vi "SW_Gen_Get_Initial_picture_Scaling_and_Cage_size.vi"(8 "Input cluster of parameters":T2={"Amount of border segments"=8, "Border segments starting angle"=0, "Amount of midfield segments"=4, "Midfield segments starting angle"=0, "Midfield segments outer radius, mm"=60, "Amount of central segments"=1, "Center segment outer radius, mm"=30, "Diameter of the cage, mm"=180, "R-gap between segments, mm"=10} {"Diameter of the cage, mm" scale=20.0..250.0}, 9 "Scale factor for outer display radius display":dbl=0.95 format="%#_13g", 10 "Background color":u32(colorbox)=13816530, 11 "Draw Area Size":cluster{"Width":dbl, "Height":dbl}={"Width"=480.0, "Height"=480.0}) -> (0 "Cluster of image geometrical and scaling parameters":T1, 3 "Zones display background":picture)   [LabVIEW 2018, in "Tracker.lvlib"]
uses:
  Tracker.lvlib
panel:
  out "Radius of displayed central segment, pix":dbl
  out "Radius of displayed midfield segments, pix":dbl
  out "Pixels per mm":dbl
  out "Radius of displayed outer segments, pix":dbl
  out "Fonts scale factor":dbl
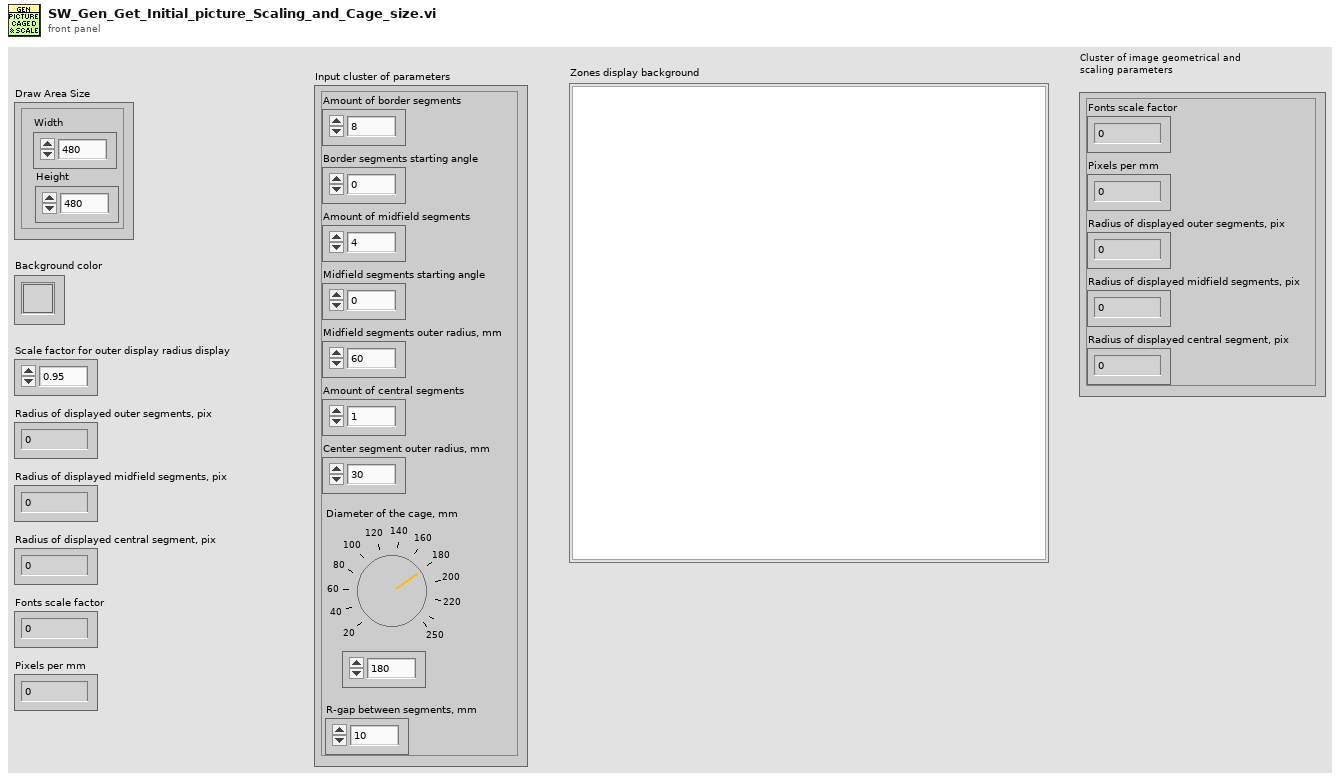
[diagram p1: front panel]
types:
  T1 = cluster{"Fonts scale factor":dbl, "Pixels per mm":dbl, "Radius of displayed outer segments, pix":dbl, "Radius of displayed midfield segments, pix":dbl, "Radius of displayed central segment, pix":dbl}
  T2 = cluster{"Amount of border segments":u8, "Border segments starting angle":i16, "Amount of midfield segments":u8, "Midfield segments starting angle":i16, "Midfield segments outer radius, mm":u16, "Amount of central segments":u8, "Center segment outer radius, mm":u16, "Diameter of the cage, mm":u16, "R-gap between segments, mm":u8}
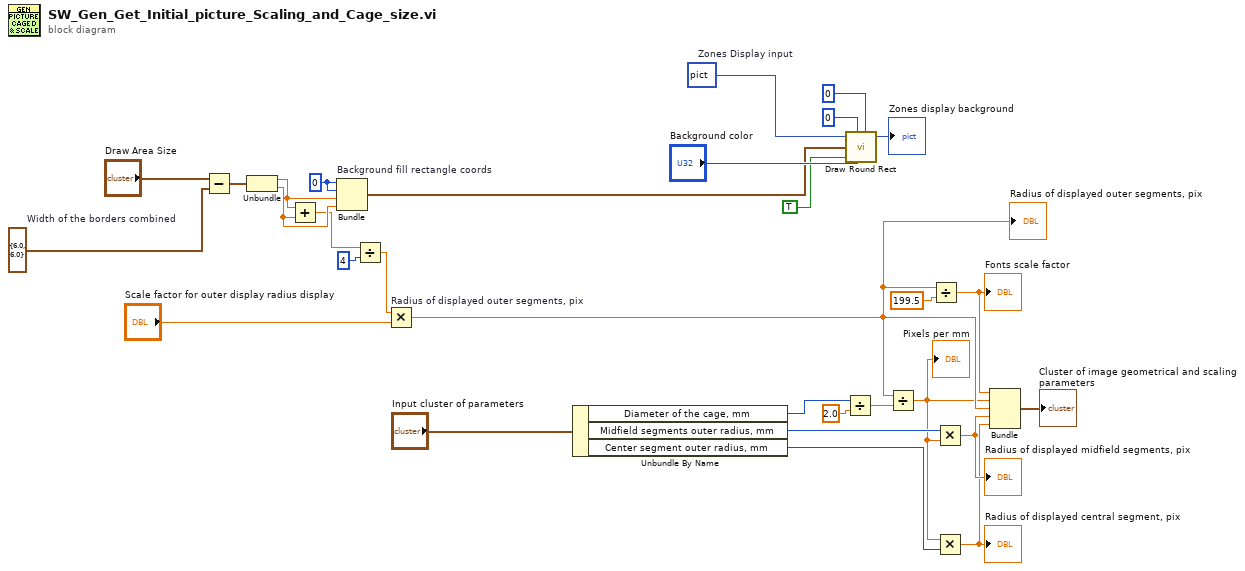
[diagram p0: block diagram]
diagram:
  w17 = cluster{"Width":dbl, "Height":dbl} {"Width"=6.0, "Height"=6.0}  # Width of the borders combined
  w28 = picture data[5B]  # Zones Display input
  w14 = 0
  n1 = Subtract(x="Draw Area Size", y=w17) -> (x-y=w15:cluster{"Width":dbl, "Height":dbl})
  n2 = Unbundle(w15) -> ("Width"=w23:dbl, "Height"=w24:dbl)
  n3 = Add(x=w23, y=w24) -> (x+y=w22:dbl)
  n4 = Bundle "Background fill rectangle coords"(w14, w14, "Width"=w23, "Height"=w24) -> (w4:cluster{i32, i32, "Width":dbl, "Height":dbl})  [unwired: 1 in]
  n5 = Divide(x=w22, y=u32 4) -> (x/y=w19:dbl)
  n6 = Multiply "Radius of displayed outer segments, pix"(x=w19, y="Scale factor for outer display radius display") -> (x*y=w8:dbl)
  "Radius of displayed outer segments, pix" <- w8
  n7 = Unbundle By Name("Input cluster of parameters") -> ("Diameter of the cage, mm"=w10:u16, "Midfield segments outer radius, mm"=w7:u16, "Center segment outer radius, mm"=w5:u16)
  n8 = Divide(x=w10, y=2.0) -> (x/y=w12:dbl)
  n9 = call <vilib>:"Draw Round Rect.vi"("picture"=w28, "oval width"=i16 0, "rect"=w4, "fill?(F)"=TRUE, "color(black)"="Background color", "oval height"=i16 0) -> ("new picture"=→"Zones display background":picture)  [unwired: 3 in]
  n10 = Divide(x=w8, y=w12) -> (x/y=w6:dbl)
  "Pixels per mm" <- w6
  n11 = Divide(x=w8, y=199.5) -> (x/y=w9:dbl)
  "Fonts scale factor" <- w9
  n12 = Multiply(x=w7, y=w6) -> (x*y=w3:dbl)
  "Radius of displayed midfield segments, pix" <- w3
  n13 = Multiply(x=w6, y=w5) -> (x*y=w2:dbl)
  "Radius of displayed central segment, pix" <- w2
  n14 = Bundle(w9, w6, w8, w3, w2) -> (→"Cluster of image geometrical and scaling parameters":cluster{dbl, dbl, dbl, dbl, dbl})  [unwired: 1 in]
